vi "N9010A_xnode_to_terms.vi"(8 "error in (no error)":errorcluster, 10 "BlockNodeState":T5 {"Draw Style" items=["FunctionBlock", "ExpressVI", "Variable", "Elemental I/O", "32x32 Icon", "FunctionBlockCompact"]; "Terminal Data"."Terminal Flags" format="%.0b"}, 11 "VI Refnum":refnum<vi>) -> (0 "error out":errorcluster, 1 "GrownTerms":string[](array[string]), 2 "Terms":T1, 3 "VI Refnum out":refnum<vi>)   [LabVIEW 2018]
uses:
  <vilib>/BlockNodeSupport/BlockNodeState.ctl
  <vilib>/BlockNodeSupport/TerminalData.ctl
  <vilib>/picture/picture.llb/imagedata.ctl
  <vilib>/XNodeSupport/XNodeTermIDPairs.ctl
  <vilib>/XNodeSupport/XNodeTermIDPair.ctl
  <vilib>/XNodeSupport/XNodeTermRef.ctl
  <vilib>/XNodeSupport/XNodeString.ctl
  <vilib>/XNodeSupport/NI_XNodeSupport.lvlib
panel:
  out "Block Diagram":refnum<vi>
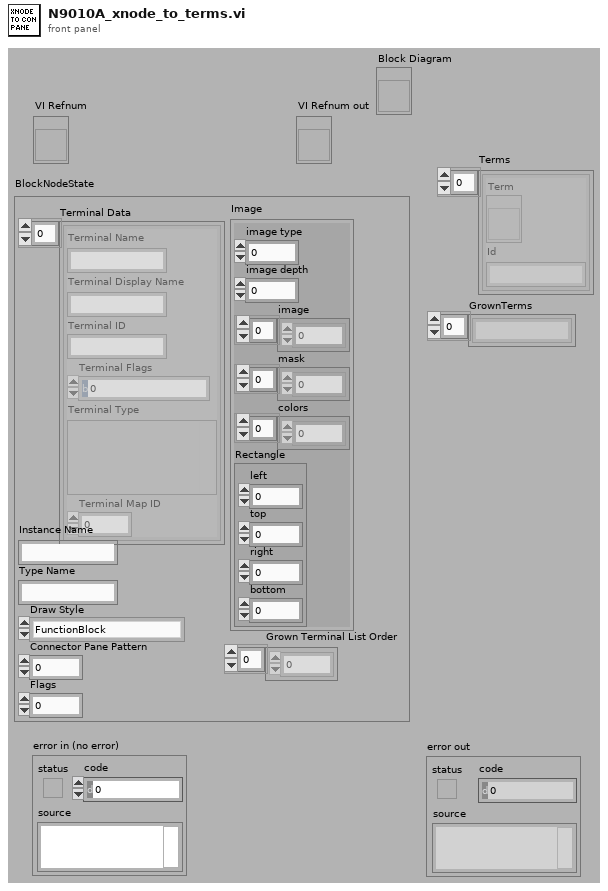
[diagram p1: front panel]
types:
  T1 = typedef "NI_XNodeSupport.lvlib/XNodeTermIDPairs.ctl" = T2[]
  T2 = typedef "NI_XNodeSupport.lvlib/XNodeTermIDPair.ctl" = cluster{"Term":T3, "Id":T4}
  T3 = typedef "NI_XNodeSupport.lvlib/XNodeTermRef.ctl" = refnum<vi>
  T4 = typedef "NI_XNodeSupport.lvlib/XNodeString.ctl" = string
  T5 = typedef "BlockNodeState.ctl" = cluster{"Terminal Data":T6[], "Instance Name":string, "Type Name":string, "Draw Style":i32, "Connector Pane Pattern":i32, "Flags":i32, "Grown Terminal List Order":i32[], "Image":T7}
  T6 = typedef "TerminalData.ctl" = cluster{"Terminal Name":string, "Terminal Display Name":string, "Terminal ID":string, "Terminal Flags":i32, "Terminal Type":variant, "Terminal Map ID":i32}
  T7 = typedef "imagedata.ctl" = cluster{"image type":i32, "image depth":i32, "image":u8[], "mask":u8[], "colors":u32[], "Rectangle":cluster{"left":i16, "top":i16, "right":i16, "bottom":i16}}
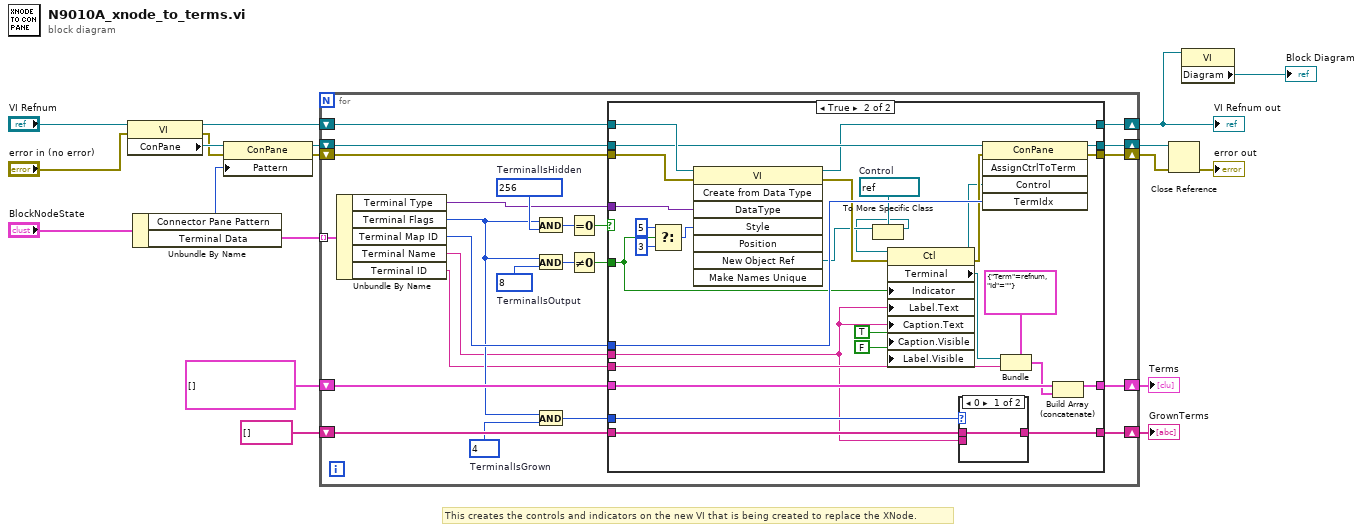
[diagram p0: block diagram]
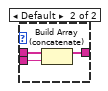
[diagram p3: hidden frame]
diagram:
  # "This creates the controls and indicators on the new VI that is being created to replace the XNode."
  n1 = property class="VI"(reference="VI Refnum", error in="error in (no error)") -> (reference out=w10:refnum<vi>, error out=w16:errorcluster, "ConPane"=w19:refnum<vi>)
  n2 = Unbundle By Name("BlockNodeState") -> ("Connector Pane Pattern"=w1:i32, "Terminal Data"=w15:T6[])
  n3 = property class="ConPane"(reference=w19, error in=w16, "Pattern"=w1) -> (reference out=w14:refnum<vi>, error out=w13:errorcluster)
  n4 = for {
    tunnel: w15 -> [w43] mode=indexing
    shift-right: [w31] -> w12
    shift-left: w14 -> [w33]
    shift-right: [w30] -> w11
    shift-left: w13 -> [w32]
    shift-right: [w36] -> w3
    shift-left: w10 -> [w37]
    shift-right: [w27] -> w6
    shift-left: T1 [] ("Terms") -> [w28]
    shift-right: [w25] -> w4
    shift-left: string[] [] -> [w26]
    w20 = 4  # TerminalIsGrown
    w41 = 8  # TerminalIsOutput
    w42 = 256  # TerminalIsHidden
    n5 = Unbundle By Name(w43) -> ("Terminal Type"=w35:variant, "Terminal Flags"=w24:i32, "Terminal Map ID"=w29:i32, "Terminal Name"=w22:string, "Terminal ID"=w23:string)
    n6 = And(x=w24, y=w42) -> (x .and. y?=w40:i32)
    n7 = And(x=w24, y=w41) -> (x .and. y?=w39:i32)
    n8 = And(x=w24, y=w20) -> (x .and. y?=w21:i32)
    n9 = Equal To 0?(x=w40) -> (x = 0?=w38:bool)
    n10 = Not Equal To 0?(x=w39) -> (x != 0?=w34:bool)
    n11 = case shown="True" w38 {
      tunnel: w37 -> [w48 w74]
      tunnel: [w48 w70] -> w36
      tunnel: w35 -> [_ w78]
      tunnel: w34 -> [_ w58]
      tunnel: w33 -> [w47 w73]
      tunnel: w32 -> [w46 w72]
      tunnel: [w47 w71] -> w31
      tunnel: [w46 w69] -> w30
      tunnel: w29 -> [_ w68]
      tunnel: w28 -> [w45 w67]
      tunnel: [w45 w66] -> w27
      tunnel: w23 -> [_ w62]
      tunnel: w26 -> [w44 w57]
      tunnel: [w44 w56] -> w25
      tunnel: w21 -> [_ w55]
      tunnel: w22 -> [_ w53]
      frame False {
      }
      frame True {
        w50 = refnum<vi> refnum  # Control
        n12 = Select(t=5, s=w58, f=3) -> (s? t:f=w75:i32)
        n13 = invoke class="VI" method="Create from Data Type"(reference=w74, error in=w72, "DataType"=w78, "Style"=w75) -> (reference out=w70:refnum<vi>, error out=w61:errorcluster, "New Object Ref"=w51:refnum<vi>)  [unwired: 4 in, 5 out]
        n14 = To More Specific Class(target class=w50, reference=w51) -> (specific class reference=w49:refnum<vi>)  [unwired: 1 in, 1 out]
        n15 = property class="Ctl"(reference=w49, error in=w61, "Indicator"=w58, "Label.Text"=w53, "Caption.Text"=w53, "Caption.Visible"=TRUE, "Label.Visible"=FALSE) -> (reference out=w59:refnum<vi>, error out=w60:errorcluster, "Terminal"=w63:refnum<vi>)
        n16 = case shown="0" w55 {
          tunnel: w57 -> [w79 w82]
          tunnel: [w79 w81] -> w56
          tunnel: w53 -> [_ w80]
          frame 0 {
          }
          frame Default {
            n17 = Build Array (concatenate)(w82, w80) -> (w81:string[])
          }
        }
        n18 = invoke class="ConPane" method="AssignCtrlToTerm"(reference=w73, error in=w60, "Control"=w59, "TermIdx"=w68) -> (reference out=w71:refnum<vi>, error out=w69:errorcluster)  [unwired: 1 in, 3 out]
        n19 = Bundle(cluster=T2 {"Term"=refnum, "Id"=""} ("Code Gen Term"), "Term"=w63, "Id"=w62) -> (w64:T2)
        n20 = Build Array (concatenate)(w67, w64) -> (w66:T1)
      }
    }
  }
  "VI Refnum out" <- w3
  "Terms" <- w6
  "GrownTerms" <- w4
  n21 = Close Reference(reference=w12, error in (no error)=w11) -> (error out=→"error out":errorcluster)
  n22 = property class="VI"(reference=w3) -> ("Diagram"=→"Block Diagram":refnum<vi>)  [unwired: 1 in, 2 out]
